vi "MongoDB.FormatObject_ID.vi"(8 "Error In":errorcluster, 11 "JSON In":string) -> (0 "Error Out":errorcluster, 3 "JSON Out":string)   [LabVIEW 2014]
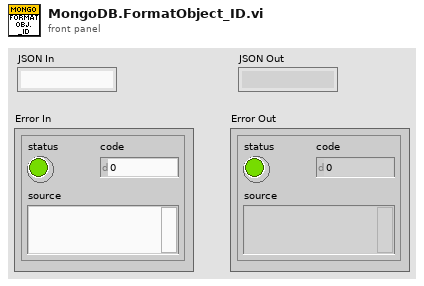
[diagram p1: front panel]
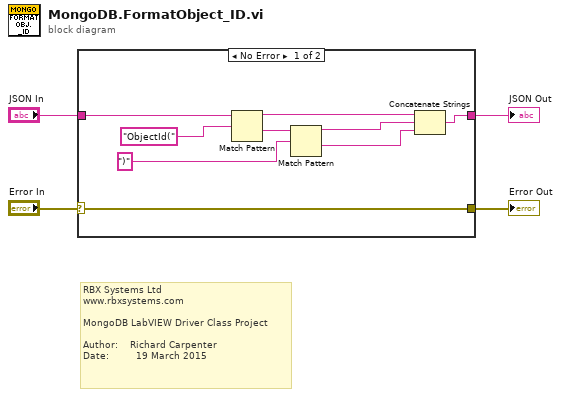
[diagram p0: block diagram]
diagram:
  # "RBX Systems Ltd\nwww.rbxsystems.com\n\nMongoDB LabVIEW Driver Class Project\n\nAuthor:    Richard Carpenter\nDate:         19 March 2015"
  n1 = case shown="No Error" "Error In" {
    selector: "Error In" -> [w5 w14]
    tunnel: [w13 w15] -> w4
    tunnel: "JSON In" -> [w7 w15]
    tunnel: [w5 w14] -> w1
    frame No Error {
      n2 = Match Pattern(string=w7, regular expression="ObjectId(" ("Result")) -> (before substring=w10:string, after substring=w8:string)  [unwired: 1 in, 2 out]
      n3 = Match Pattern(string=w8, regular expression=")" ("Result")) -> (before substring=w11:string, after substring=w12:string)  [unwired: 1 in, 2 out]
      n4 = Concatenate Strings(w10, w11, w12) -> (w13:string)
    }
    frame Error {
    }
  }
  "JSON Out" <- w4
  "Error Out" <- w1
